vi "Read Measurement (Effective Temperature).vi"(8 "error in (no error)":errorcluster, 9 "Maximum Time (20000 ms)":i32=20000, 10 "Measurement Type (0: Corrected)":u16(ring) items=["Corrected", "Uncorrected"], 11 "VISA resource name":refnum<visa-resource-name>) -> (0 "error out":errorcluster, 2 "Effective Temperature Results (K)":dbl[](array[numeric]), 3 "VISA resource name out":refnum<visa-resource-name>)   [LabVIEW 2014, in "Agilent ESA PSA Series.lvlib"]
doc: "Stops the present measurement and sets up the instrument for a Noise Figure, Effective Temperature measurement.\n\nAfter the data are valid, the result is returned for the specified measurement. These are the settings and units that conform to the measurement specific standard.\n\n- Stops the current measurement and does not reset the measurement to the factory defaults. \n\n- Initiates the measurement and puts valid data into the output buffer. If a measurement other than the current one is specified, the instrument will switch to that measurement before it initiates the measurement and returns results.\n\n- Waits until the measurement is complete before returning results.\n\n<B>Note:</B>\n\nThis VI is only valid for the Noise Figure functionality of the Noise Figure personality."
uses:
  Agilent ESA PSA Series.lvlib
  Fetch Measurement (Effective Temperature).vi
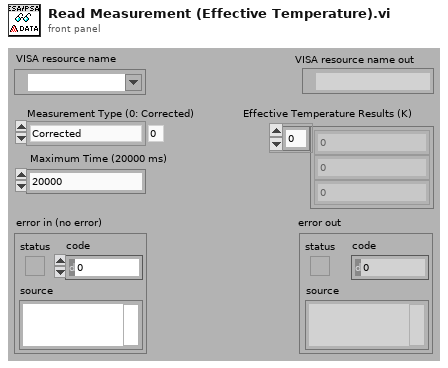
[diagram p1: front panel]
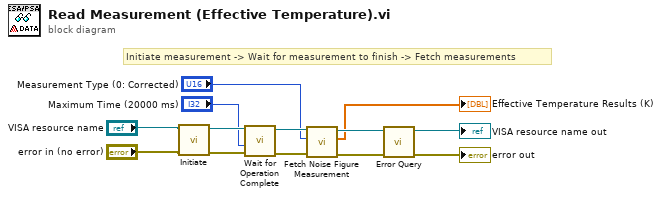
[diagram p0: block diagram]
diagram:
  # "Initiate measurement -> Wait for measurement to finish -> Fetch measurements"
  n1 = call "Initiate.vi"("error in (no error)"="error in (no error)", "VISA resource name"="VISA resource name") -> ("error out"=w10:errorcluster, "VISA resource name out"=w11:refnum<visa-resource-name>)  [unwired: 8 in]
  n2 = call "Wait for Operation Complete.vi"("error in (no error)"=w10, "Maximum Time (10000ms)"="Maximum Time (20000 ms)", "VISA resource name"=w11) -> ("error out"=w6:errorcluster, "VISA resource name out"=w7:refnum<visa-resource-name>)  [unwired: 7 in]
  n3 = call-poly "Fetch Noise Figure Measurement.vi"("error in (no error)"=w6, "Measurement Type (0: Corrected)"="Measurement Type (0: Corrected)", "VISA resource name"=w7) -> ("error out"=w4:errorcluster, "Effective Temperature Results (K)"=→"Effective Temperature Results (K)":dbl[], "VISA resource name out"=w5:refnum<visa-resource-name>)  [unwired: 6 in]
  n4 = call "Error Query.vi"("error in (no error)"=w4, "VISA resource name"=w5) -> ("error out"=→"error out":errorcluster, "VISA resource name out"=→"VISA resource name out":refnum<visa-resource-name>)  [unwired: 6 in, 2 out]
